vi "Generate All VI HTML Documentation.vi"(5 "Images Destination":path=path "", 6 "Requirement":string="Labstache", 7 "HTML Destination":path=path "", 8 "Error In":errorcluster, 11 "Source In":path=path "") -> (0 "Error Out":errorcluster, 3 "Source Out":path)   [LabVIEW 2018, in "Scripts.lvlib"]
uses:
  Scripts.lvlib
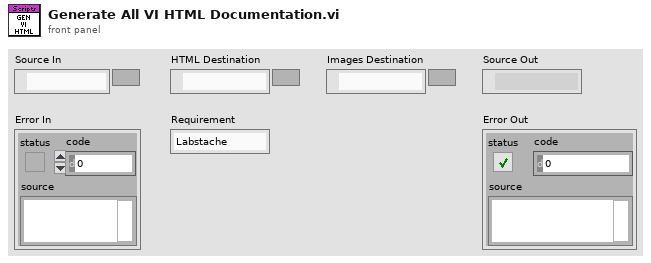
[diagram p1: front panel]
types:
  T1 = enum32{"invalid VI type", "Standard VI", "Control VI", "Global VI", "Polymorphic VI", "Configuration VI", "SubSystem", "Facade VI", "Method VI", "Statechart Diagram VI"}
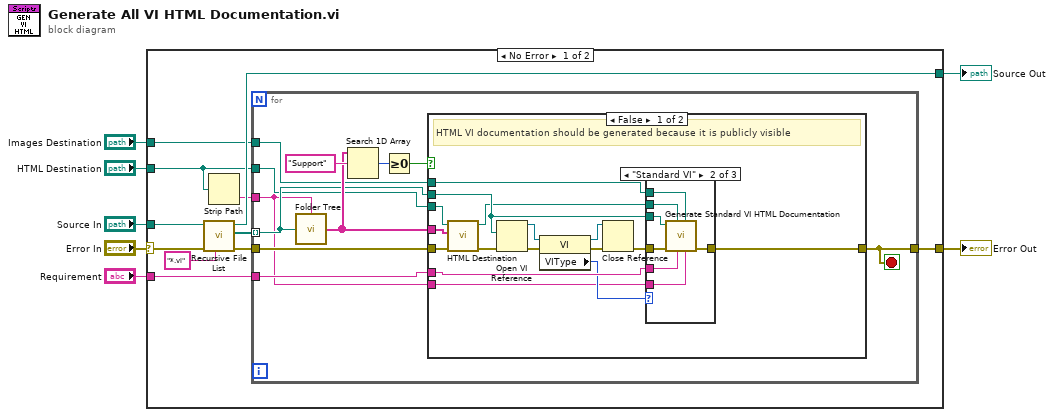
[diagram p0: block diagram]
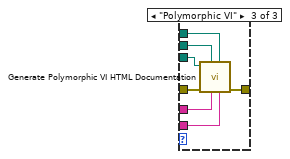
[diagram p3: hidden frame]
diagram:
  n1 = case shown="No Error" "Error In" {
    selector: "Error In" -> [w13 w63]
    tunnel: [w15 w63] -> w7
    tunnel: "Requirement" -> [w14 _]
    tunnel: "HTML Destination" -> [w10 _]
    tunnel: "Source In" -> [w12 w62]
    tunnel: [w11 w62] -> w2
    tunnel: "Images Destination" -> [w8 _]
    frame No Error {
      n2 = call <vilib>:"Recursive File List.vi"("pattern"="*.vi", "error in (no error)"=w13, "Folder Path"=w12) -> ("error out"=w16:errorcluster, "All Files in Dir"=w17:path[], "dup Folder Path"=w11:path)  [unwired: 4 in, 2 out]
      n3 = Strip Path(path=w10) -> (name=w9:string)  [unwired: 1 out]
      n4 = for {
        tunnel: w17 -> [w23] mode=indexing
        tunnel: w16 -> [w25]
        tunnel: w9 -> [w21]
        tunnel: [w24] -> w15
        tunnel: w14 -> [w22]
        tunnel: w10 -> [w20]
        tunnel: w8 -> [w19]
        stop <- w24 stop-if-true
        n5 = call "Folder Tree.vi"("File"=w23, "Root Folder Name"=w21) -> ("Hierarchy Folders"=w26:string[])
        n6 = Search 1D Array(1D array=w26, element="Support") -> (index of element=w28:i32)  [unwired: 1 in]
        n7 = Greater Or Equal To 0?(x=w28) -> (x >= 0?=w27:bool)
        n8 = case shown="False" w27 {
          tunnel: w26 -> [w44 _]
          tunnel: w25 -> [w45 w61]
          tunnel: [w43 w61] -> w24
          tunnel: w23 -> [w37 _]
          tunnel: w22 -> [w42 _]
          tunnel: w21 -> [w34 _]
          tunnel: w20 -> [w33 _]
          tunnel: w19 -> [w30 _]
          frame False {
            # "HTML VI documentation should be generated because it is publicly visible"
            n9 = call "HTML Destination.vi"("Error In"=w45, "Hierarchy Folders"=w44, "Root Destination"=w33) -> ("Error Out"=w41:errorcluster, "HTML Destination"=w36:path)  [unwired: 7 in]
            n10 = Open VI Reference(vi path=w37, error in (no error)=w41) -> (vi reference=w40:refnum<vi>, error out=w39:errorcluster)  [unwired: 4 in]
            n11 = property class="VI"(reference=w40, error in=w39) -> (reference out=w31:refnum<vi>, error out=w32:errorcluster, "VIType"=w38:T1)
            n12 = Close Reference(reference=w31, error in (no error)=w32) -> (error out=w35:errorcluster)
            n13 = case shown="\"Standard VI\"" w38 {
              tunnel: [w46 w53 w59] -> w43
              tunnel: w42 -> [_ w50 w56]
              tunnel: w37 -> [_ w52 w60]
              tunnel: w36 -> [_ w48 w57]
              tunnel: w35 -> [w46 w51 w58]
              tunnel: w34 -> [_ w49 w55]
              tunnel: w30 -> [_ w47 w54]
              frame "invalid VI type", Default {
              }
              frame "Standard VI" {
                n14 = call "Generate Standard VI HTML Documentation.vi"("Root Folder Name"=w49, "Images Destination"=w47, "Requirement"=w50, "Destination"=w48, "Error In"=w51, "VI"=w52) -> ("Error Out"=w53:errorcluster)  [unwired: 5 in]
              }
              frame "Polymorphic VI" {
                n15 = call "Generate Polymorphic VI HTML Documentation.vi"("Root Folder Name"=w55, "Images Destination"=w54, "Requirement"=w56, "Destination"=w57, "Error In"=w58, "VI"=w60) -> ("Error Out"=w59:errorcluster)  [unwired: 5 in]
              }
            }
          }
          frame True {
            # "Is a private VI that does not need VI documentation generated"
          }
        }
      }
    }
    frame Error {
    }
  }
  "Error Out" <- w7
  "Source Out" <- w2
